vi "AG-UC2-scan.vi"() -> ()   [LabVIEW 2012]
uses:
  D:/workspace/GitHub/LVsolis/lib/AgilisCmdLib.dll
  lib/AgilisCmdLib.dll
panel:
  in  "Set zero":bool
  out "Position":u64
  in  "Exit":bool
  out "Stop":bool
  out "Scan":bool
  in  "Cancel":bool
  in  "Scan":bool
  in  "Step number":dbl
  in  "Step size":i64
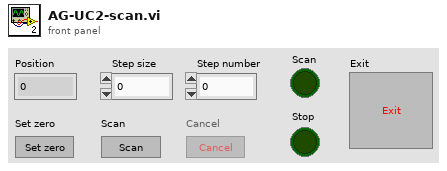
[diagram p1: front panel]
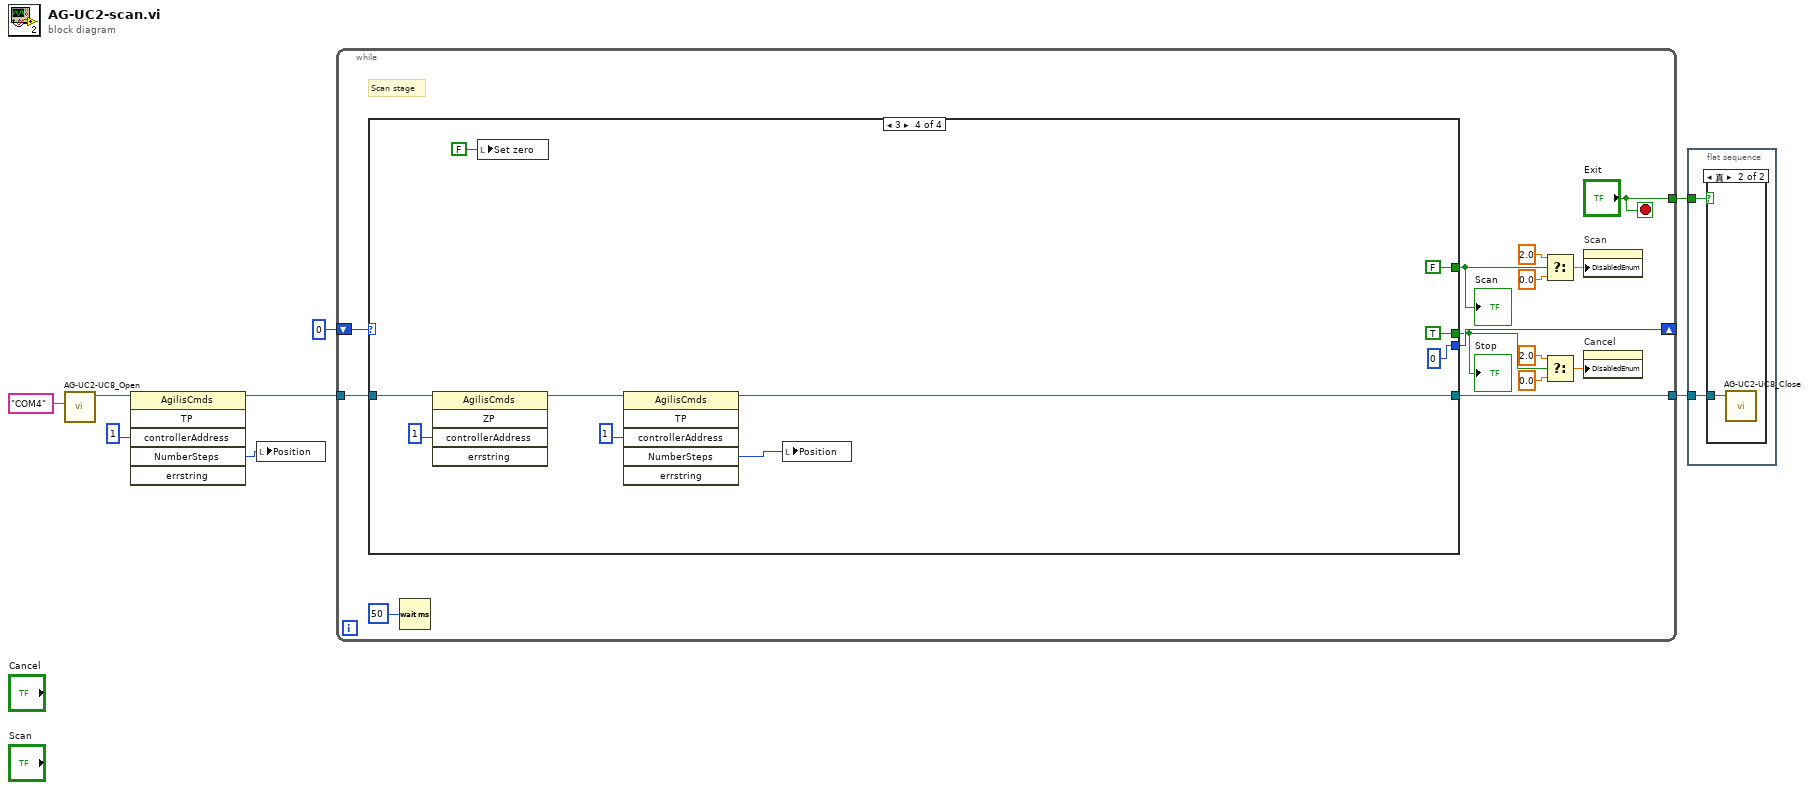
[diagram p0: block diagram]
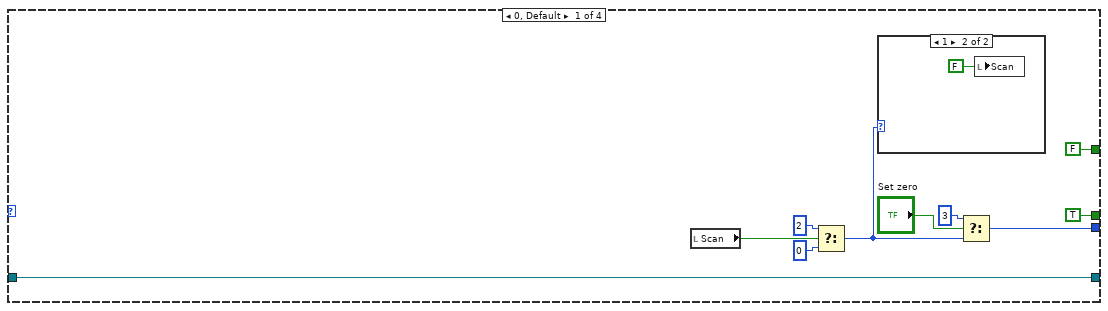
[diagram p3: hidden frame]
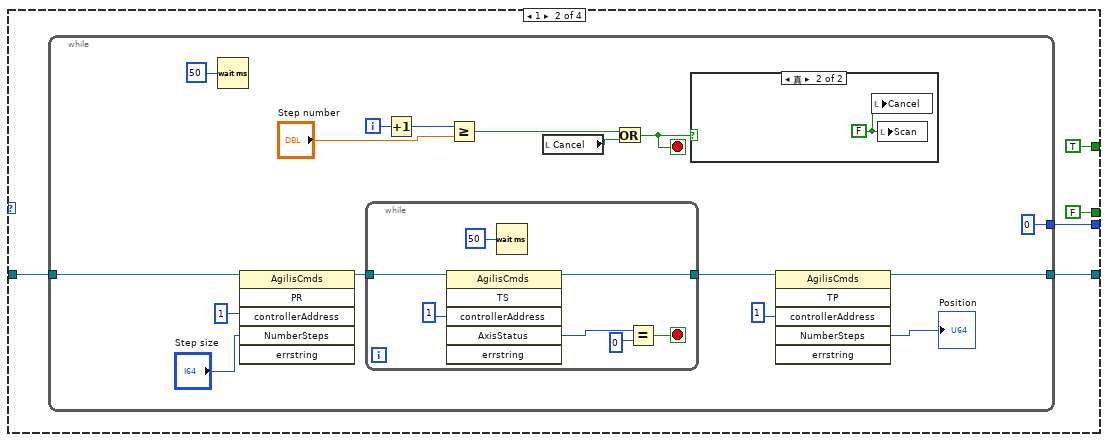
[diagram p5: hidden frame]
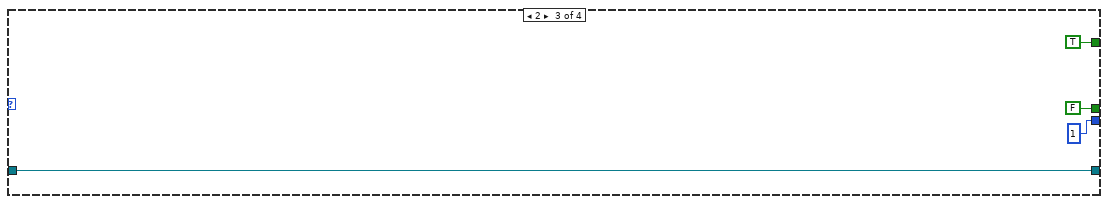
[diagram p7: hidden frame]
diagram:
  n1 = call "AG-UC2-UC8_Open.vi"("Instrument Key IN"="COM4") -> ("AG-UC2-UC8 Reference"=w6:refnum<k24>)  [unwired: 3 in, 3 out]
  n2 = invoke class="AgilisCmds" method="TP"(reference=w6, "controllerAddress"=1) -> (reference out=w1:refnum<k24>, "NumberSteps"=w4:i32)  [unwired: 4 in, 4 out]
  n3 = local write "Position"(w4) -> ()
  n4 = while {
    shift-right: [w21] -> _
    shift-left: 0 -> [w22]
    tunnel: w1 -> [w11]
    tunnel: ["Exit"] -> w3
    tunnel: [w9] -> w2
    stop <- "Exit" stop-if-true
    # "Scan stage"
    n5 = case shown="3" w22 {
      tunnel: [w23 w38 1 0 ("t")] -> w21
      tunnel: [TRUE ("Scan") FALSE FALSE TRUE ("Scan")] -> w19
      tunnel: [FALSE ("Scan") TRUE TRUE FALSE ("Scan")] -> w20
      tunnel: w11 -> [w27 w35 w63 w73]
      tunnel: [w27 w34 w63 w68] -> w9
      frame 0, Default {
        n6 = local read "Scan"() -> (w32:bool)
        n7 = Select(t=2, s=w32, f=0) -> (s? t:f=w24:i32)
        n8 = case shown="1" w24 {
          frame 0, Default {
          }
          frame 1 {
            n9 = local write "Scan"(FALSE ("Scan")) -> ()
          }
        }
        n10 = Select(t=u8 3, s="Set zero", f=w24) -> (s? t:f=w23:i32)
      }
      frame 1 {
        n11 = while {
          tunnel: [0] -> w38
          tunnel: w35 -> [w46]
          tunnel: [w41] -> w34
          i -> [w48]
          stop <- w50 stop-if-true
          n12 = Wait (ms)(milliseconds to wait=u32 50 ("等待时间（毫秒）")) -> ()  [unwired: 1 out]
          n13 = invoke class="AgilisCmds" method="PR"(reference=w46, "controllerAddress"=1, "NumberSteps"="Step size") -> (reference out=w40:refnum<k24>)  [unwired: 3 in, 5 out]
          n14 = while {
            tunnel: w40 -> [w60]
            tunnel: [w59] -> w39
            stop <- w55 stop-if-true
            n15 = invoke class="AgilisCmds" method="TS"(reference=w60, "controllerAddress"=1) -> (reference out=w59:refnum<k24>, "AxisStatus"=w57:i32)  [unwired: 4 in, 4 out]
            n16 = Wait (ms)(milliseconds to wait=u32 50 ("等待时间（毫秒）")) -> ()  [unwired: 1 out]
            n17 = Equal?(x=w57, y=0) -> (x = y?=w55:bool)
          }
          n18 = Increment(x=w48) -> (x+1=w47:i32)
          n19 = Greater Or Equal?(x=w47, y="Step number") -> (x >= y?=w53:bool)
          n20 = local read "Cancel"() -> (w54:bool)
          n21 = Or(x=w53, y=w54) -> (x .or. y?=w50:bool)
          n22 = case shown="真" w50 {
            frame False {
            }
            frame True {
              w62 = FALSE
              n23 = local write "Cancel"(w62) -> ()
              n24 = local write "Scan"(w62) -> ()
            }
          }
          n25 = invoke class="AgilisCmds" method="TP"(reference=w39, "controllerAddress"=1) -> (reference out=w41:refnum<k24>, "NumberSteps"=→"Position":i32)  [unwired: 4 in, 4 out]
        }
      }
      frame 2 {
      }
      frame 3 {
        n26 = invoke class="AgilisCmds" method="ZP"(reference=w73, "controllerAddress"=1) -> (reference out=w72:refnum<k24>)  [unwired: 3 in, 4 out]
        n27 = local write "Set zero"(FALSE ("Set zero")) -> ()
        n28 = invoke class="AgilisCmds" method="TP"(reference=w72, "controllerAddress"=1) -> (reference out=w68:refnum<k24>, "NumberSteps"=w71:i32)  [unwired: 4 in, 4 out]
        n29 = local write "Position"(w71) -> ()
      }
    }
    "Scan" <- w20
    "Stop" <- w19
    n30 = Wait (ms)(milliseconds to wait=u32 50 ("等待时间（毫秒）")) -> ()  [unwired: 1 out]
    n31 = Select(t=2.0, s=w20, f=0.0) -> (s? t:f=w13:dbl)
    n32 = Select(t=2.0, s=w19, f=0.0) -> (s? t:f=w12:dbl)
    n33 = property on="Scan" class="Bool (严格)"("DisabledEnum"=w13) -> ()  [unwired: 2 in, 2 out]
    n34 = property on="Cancel" class="Bool (严格)"("DisabledEnum"=w12) -> ()  [unwired: 2 in, 2 out]
  }
  n35 = flat-sequence {
    tunnel: w3 -> [w78]
    tunnel: w2 -> [w77]
    frame #0 {
      n36 = case shown="真" w78 {
        tunnel: w77 -> [_ w79]
        frame False {
        }
        frame True {
          n37 = call "AG-UC2-UC8_Close.vi"("AG-UC2-UC8 Reference"=w79) -> ()  [unwired: 3 in, 2 out]
        }
      }
    }
  }
